vi "sevensegment.vi"() -> ()   [LabVIEW 2017]
panel:
  out "element 8":bool
  out "element 7":bool
  out "element 6":bool
  out "element 5":bool
  out "element 4":bool
  out "element 3":bool
  out "element 2":bool
  out "element":bool
  in  "Input Number":dbl
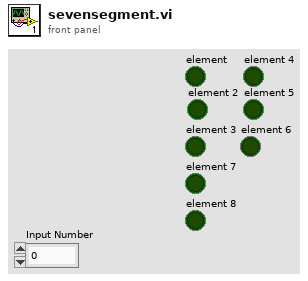
[diagram p1: front panel]
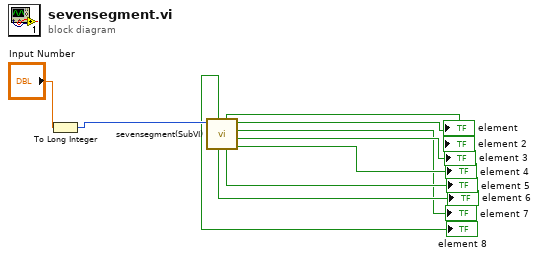
[diagram p0: block diagram]
diagram:
  n1 = To Long Integer(number="Input Number") -> (32bit integer=w9:i32)
  n2 = call "sevensegment(SubVI).vi"("Numeric"=w9) -> ("Boolean 5"=→"element 4":bool, "Boolean 6"=→"element 3":bool, "Boolean 2"=→"element 7":bool, "Boolean 7"=→"element 2":bool, "Boolean 4"=→"element 5":bool, "Boolean 8"=→"element":bool, "Boolean 3"=→"element 6":bool, "Boolean"=→"element 8":bool)  [unwired: 3 in]
